vi "Post-Install Custom Action.vi"(10 "Variant":variant) -> (0 "error out":errorcluster)   [LabVIEW 2020]
uses:
  <vilib>/zip/NI_Unzip.lvlib
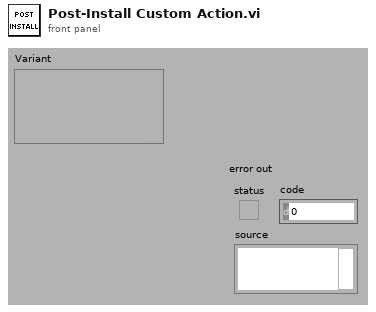
[diagram p1: front panel]
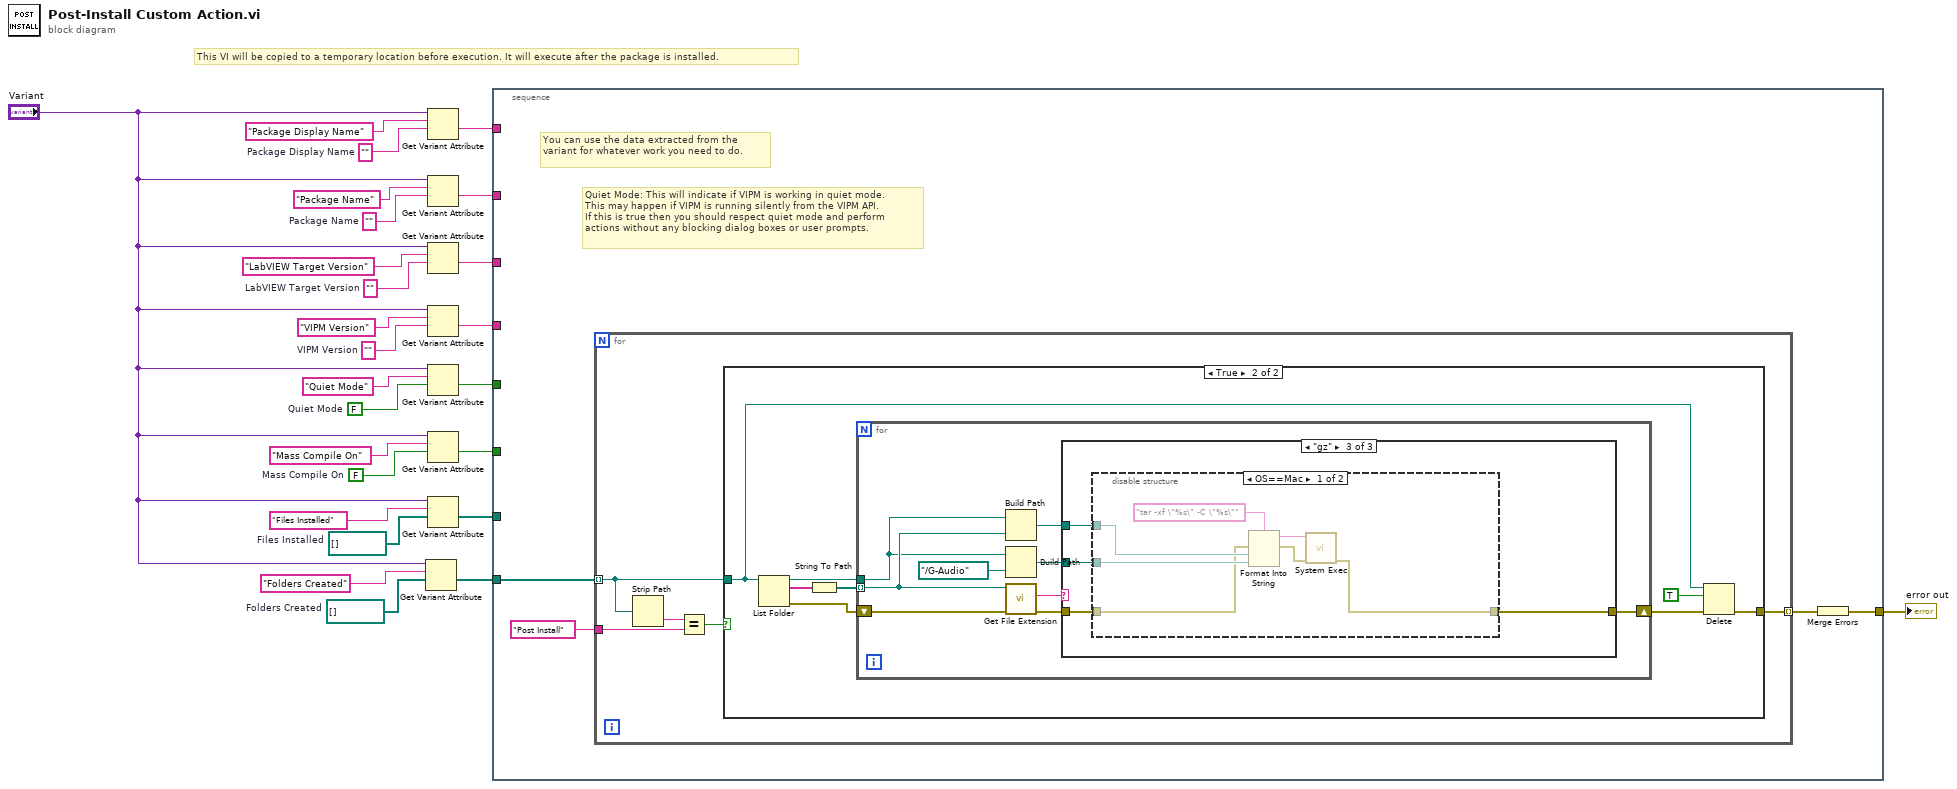
[diagram p0: block diagram]
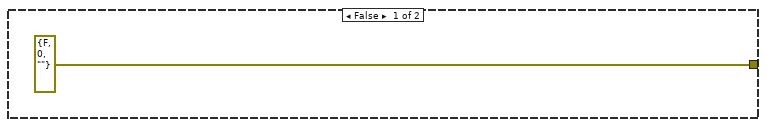
[diagram p2: hidden frame]
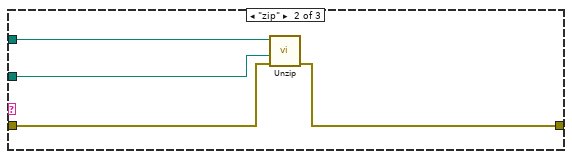
[diagram p4: hidden frame]
diagram:
  w2 = path[] []  # Folders Created
  w3 = path[] []  # Files Installed
  w9 = FALSE  # Mass Compile On
  w10 = ""  # Package Display Name
  w17 = FALSE  # Quiet Mode
  w20 = ""  # VIPM Version
  w22 = ""  # LabVIEW Target Version
  w24 = ""  # Package Name
  # "This VI will be copied to a temporary location before execution. It will execute after the package is installed."
  n1 = Get Variant Attribute(Variant="Variant", name="Folders Created", default value (empty Variant)=w2) -> (value=w7:path[])  [unwired: 1 in, 3 out]
  n2 = Get Variant Attribute(Variant="Variant", name="Package Display Name", default value (empty Variant)=w10) -> (value=w16:string)  [unwired: 1 in, 3 out]
  n3 = Get Variant Attribute(Variant="Variant", name="Package Name", default value (empty Variant)=w24) -> (value=w15:string)  [unwired: 1 in, 3 out]
  n4 = Get Variant Attribute(Variant="Variant", name="LabVIEW Target Version", default value (empty Variant)=w22) -> (value=w14:string)  [unwired: 1 in, 3 out]
  n5 = Get Variant Attribute(Variant="Variant", name="VIPM Version", default value (empty Variant)=w20) -> (value=w13:string)  [unwired: 1 in, 3 out]
  n6 = Get Variant Attribute(Variant="Variant", name="Quiet Mode", default value (empty Variant)=w17) -> (value=w12:bool)  [unwired: 1 in, 3 out]
  n7 = Get Variant Attribute(Variant="Variant", name="Mass Compile On", default value (empty Variant)=w9) -> (value=w11:bool)  [unwired: 1 in, 3 out]
  n8 = Get Variant Attribute(Variant="Variant", name="Files Installed", default value (empty Variant)=w3) -> (value=w6:path[])  [unwired: 1 in, 3 out]
  n9 = stacked-sequence {
    tunnel: w16 -> [_]
    tunnel: w15 -> [_]
    tunnel: w14 -> [_]
    tunnel: w13 -> [_]
    tunnel: w12 -> [_]
    tunnel: w11 -> [_]
    tunnel: w6 -> [_]
    tunnel: w7 -> [w30]
    tunnel: [w28] -> w1
    frame #0 {
      # "Quiet Mode: This will indicate if VIPM is working in quiet mode.\nThis may happen if VIPM is running silently from the VIPM API.\nIf this is true then you should respect quiet mode and perform\nactions without any blocking dialog boxes or user prompts."
      # "You can use the data extracted from the variant for whatever work you need to do."
      n10 = for {
        tunnel: w30 -> [w33] mode=indexing
        tunnel: "Post Install" ("y") -> [w35]
        tunnel: [w32] -> w29 mode=indexing
        n11 = Strip Path(path=w33) -> (name=w31:string)  [unwired: 1 out]
        n12 = Equal?(x=w31, y=w35) -> (x = y?=w34:bool)
        n13 = case shown="True" w34 {
          tunnel: w33 -> [_ w38]
          tunnel: [errorcluster {"status"=FALSE, "code"=0, "source"=""} ("error out") w39] -> w32
          frame False {
          }
          frame True {
            n14 = List Folder(path=w38) -> (path out=w42:path, filenames=w44:string[], error out=w41:errorcluster)  [unwired: 3 in, 1 out]
            n15 = String To Path(string=w44) -> (path=w43:path[])
            n16 = for {
              tunnel: w43 -> [w53] mode=indexing
              tunnel: w42 -> [w46]
              shift-right: [w48] -> w40
              shift-left: w41 -> [w50]
              n17 = Build Path(base path=w46, name or relative path=w53) -> (appended path=w51:path)
              n18 = Build Path(base path=w46, name or relative path=path "../G-Audio" ("Target directory (same as Zip file if empty)")) -> (appended path=w45:path)
              n19 = call <vilib>:"Get File Extension.vi"("error in (no error)"=w50, "file"=w53) -> ("error out"=w49:errorcluster, "lowercase file extension"=w52:string)  [unwired: 5 in, 3 out]
              n20 = case shown="\"gz\"" w52 {
                tunnel: w51 -> [_ w58 w60]
                tunnel: w49 -> [w54 w57 w61]
                tunnel: [w54 w56 w62] -> w48
                tunnel: w45 -> [_ w55 w59]
                frame Default {
                }
                frame "zip" {
                  n21 = call <vilib>:"Unzip.vi"("error in (no error)"=w57, "Target directory (same as Zip file if empty)"=w55, "Zip file"=w58) -> ("error out"=w56:errorcluster)  [unwired: 6 in, 2 out]
                }
                frame "gz" {
                  n22 = disable-structure shown="OS==Mac" {
                    disable-tunnel: [w69 w70] -> w62
                    disable-tunnel: w61 -> [w64 w70]
                    disable-tunnel: w60 -> [w67 _]
                    disable-tunnel: w59 -> [w66 _]
                    frame condition #0 {
                      n23 = Format Into String(format string="tar -xf \"%s\" -C \"%s\"" ("command line"), error in=w64, w67, w66) -> (resulting string=w65:string, error out=w63:errorcluster)  [unwired: 1 in]
                      n24 = call <vilib>:"System Exec.vi"("error in (no error)"=w63, "command line"=w65) -> ("error out"=w69:errorcluster)  [unwired: 6 in, 3 out]
                    }
                    frame condition #1 (active) {
                    }
                  }
                }
              }
            }
            n25 = Delete(path (use dialog)=w38, entire hierarchy (F)=TRUE, error in=w40) -> (error out=w39:errorcluster)  [unwired: 2 in, 2 out]
          }
        }
      }
      n26 = Merge Errors(w29) -> (w28:errorcluster)
    }
  }
  "error out" <- w1
